vi "LSCI_4-28.vi"() -> ()   [LabVIEW 2019]
uses:
  <resource>/objmgr/daqmx.rc
  <vilib>/DAQmx/configure/timing.llb/DAQmx Timing (Sample Clock).vi
  <vilib>/DAQmx/create/channels.llb/DAQmx Create Channel (AO-Voltage-Basic).vi
  Settings.ctl
  <vilib>/DAQmx/write.llb/DAQmx Write (Digital 1D U32 1Chan NSamp).vi
  <vilib>/DAQmx/configure/trigger.llb/DAQmx Start Trigger (Digital Edge).vi
  <vilib>/DAQmx/write.llb/DAQmx Write (Analog DBL 1Chan 1Samp).vi
  <vilib>/DAQmx/read.llb/DAQmx Read (Counter DBL 1Chan 1Samp).vi
  <vilib>/DAQmx/create/channels.llb/DAQmx Create Channel (CI-Count Edges).vi
  <vilib>/DAQmx/create/channels.llb/DAQmx Create Channel (CO-Pulse Generation-Time).vi
  <vilib>/DAQmx/write.llb/DAQmx Write (Analog Wfm 1Chan NSamp).vi
  <vilib>/DAQmx/create/channels.llb/DAQmx Create Channel (DO-Digital Output).vi
  Control 2.ctl
panel:
  out "path":path=path "D:/Haad/v1.avi1.avi"
  in  "AVI Path 2":path=path "D:/Haad/v1.avi"
  in  "Trigger":bool
  in  "Color vs Monochrome":string="Y800 (720x540)"
  in  "ICImagingControl":refnum<k7>(container)
  in  "Grab":bool
  in  "Stop":bool
  in  "AOM Voltage":dbl=0.135 format="%0.3f"
  out "String 7":string="AOM Settings"
  out "String 6":string="Stroke Settings"
  out "String 5":string="Intrinsic Imaging"
  in  "LED 625 nm":bool
  in  "LED 580 nm":bool
  out "Trial #":i32=1
  out "Frames acquired":dbl=569.0 format="%0.2f"
  out "Number of Samples (Total)":dbl=10000.0
  out "Period (ms)":dbl=7.0
  out "String 4":string="Experimental Summary"
  out "String 3":string="Stimulation Control"
  out "String 2":string="Sequence Control"
  out "String":string="Trials Control"
  in  "Strength (V)":dbl=10.0
  in  "# of stimulations":i32=2
  in  "Delay (ms)":dbl=35.0
  in  "Width of pulse (ms)":dbl=70.0
  in  "# of Sequences":dbl=100.0
  in  "Delay End (ms)":i32=51
  in  "Sampling Rate (Hz)":T1=100000.0 format="%#_9f"
  in  "Frames/Seq":i32=7
  in  "Exposure Width (ms)":T1=5.0 format="%#_9f"
  in  "Time Between (ms)":T2=2.0 format="%#_9f"
  in  "Pre-stimulus Time":dbl=5.0 format="%.6f"
  in  "Time b/w Trials (s)":dbl=5.0 caption="Delay Time (s)"
  in  "# Trials":i32=2
  in  "Time domain signal":enum32{"Trigger Sequence", "Stimulation pulse"}(tab)=enum."Stimulation pulse"
  out "LSCI Sequence":cluster{i32, dbl, dbl[]}(graph)={0, 1e-05, array[10000 elements]}
  out "Whisker Stimulus Pulse":cluster{dbl[], dbl[]}(graph)
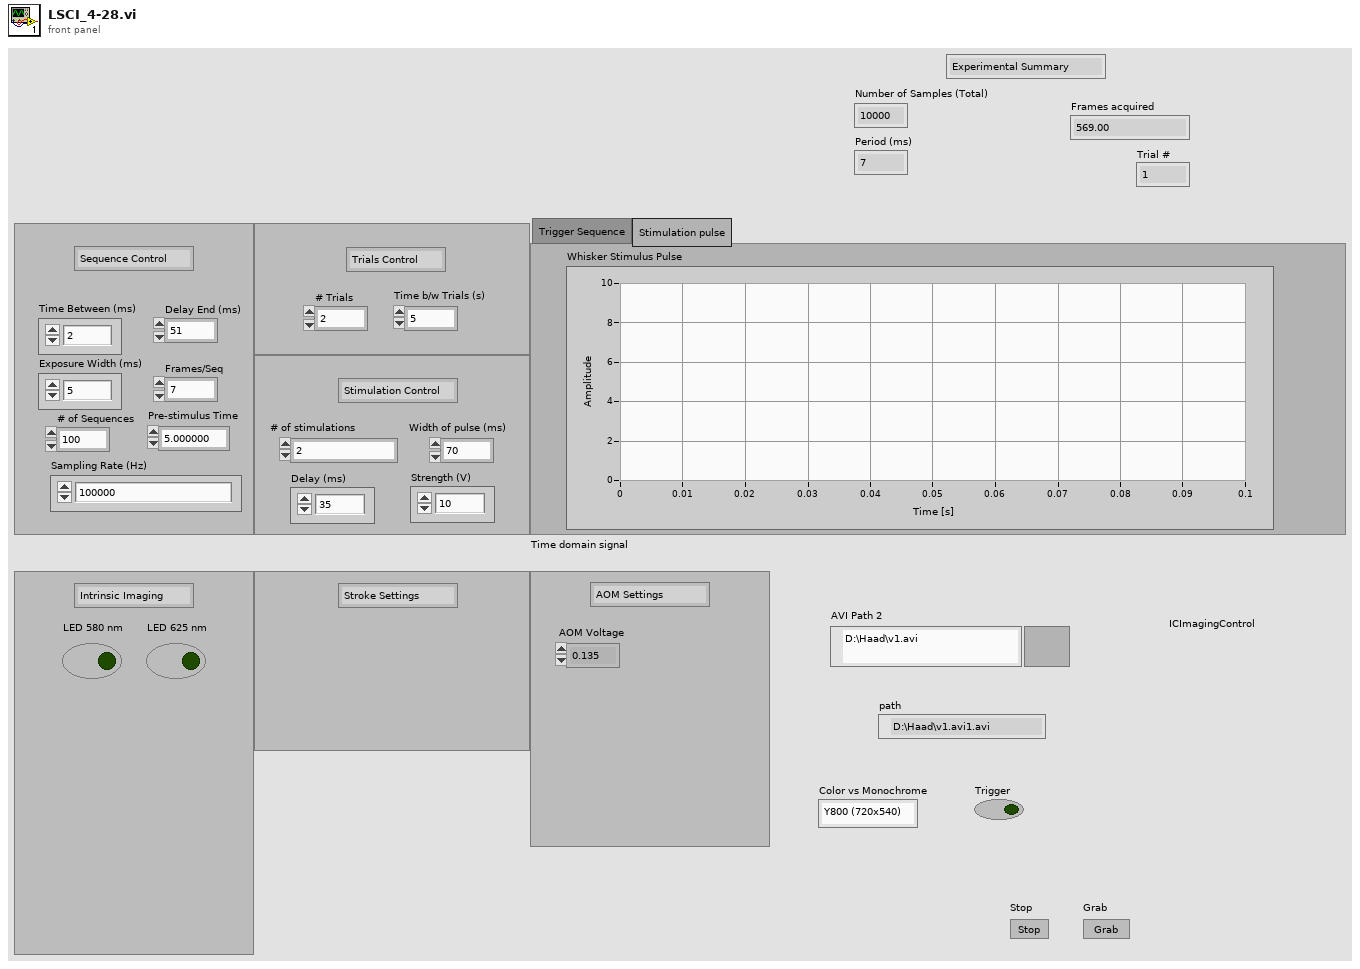
[diagram p1: front panel]
types:
  T1 = typedef "Settings.ctl" = dbl
  T2 = typedef "Control 2.ctl" = dbl
  T3 = typedef "IMAQ AVI2 Refnum.ctl" = refnum<k20>
  T4 = typedef "IMAQ Image.ctl" = refnum<image>
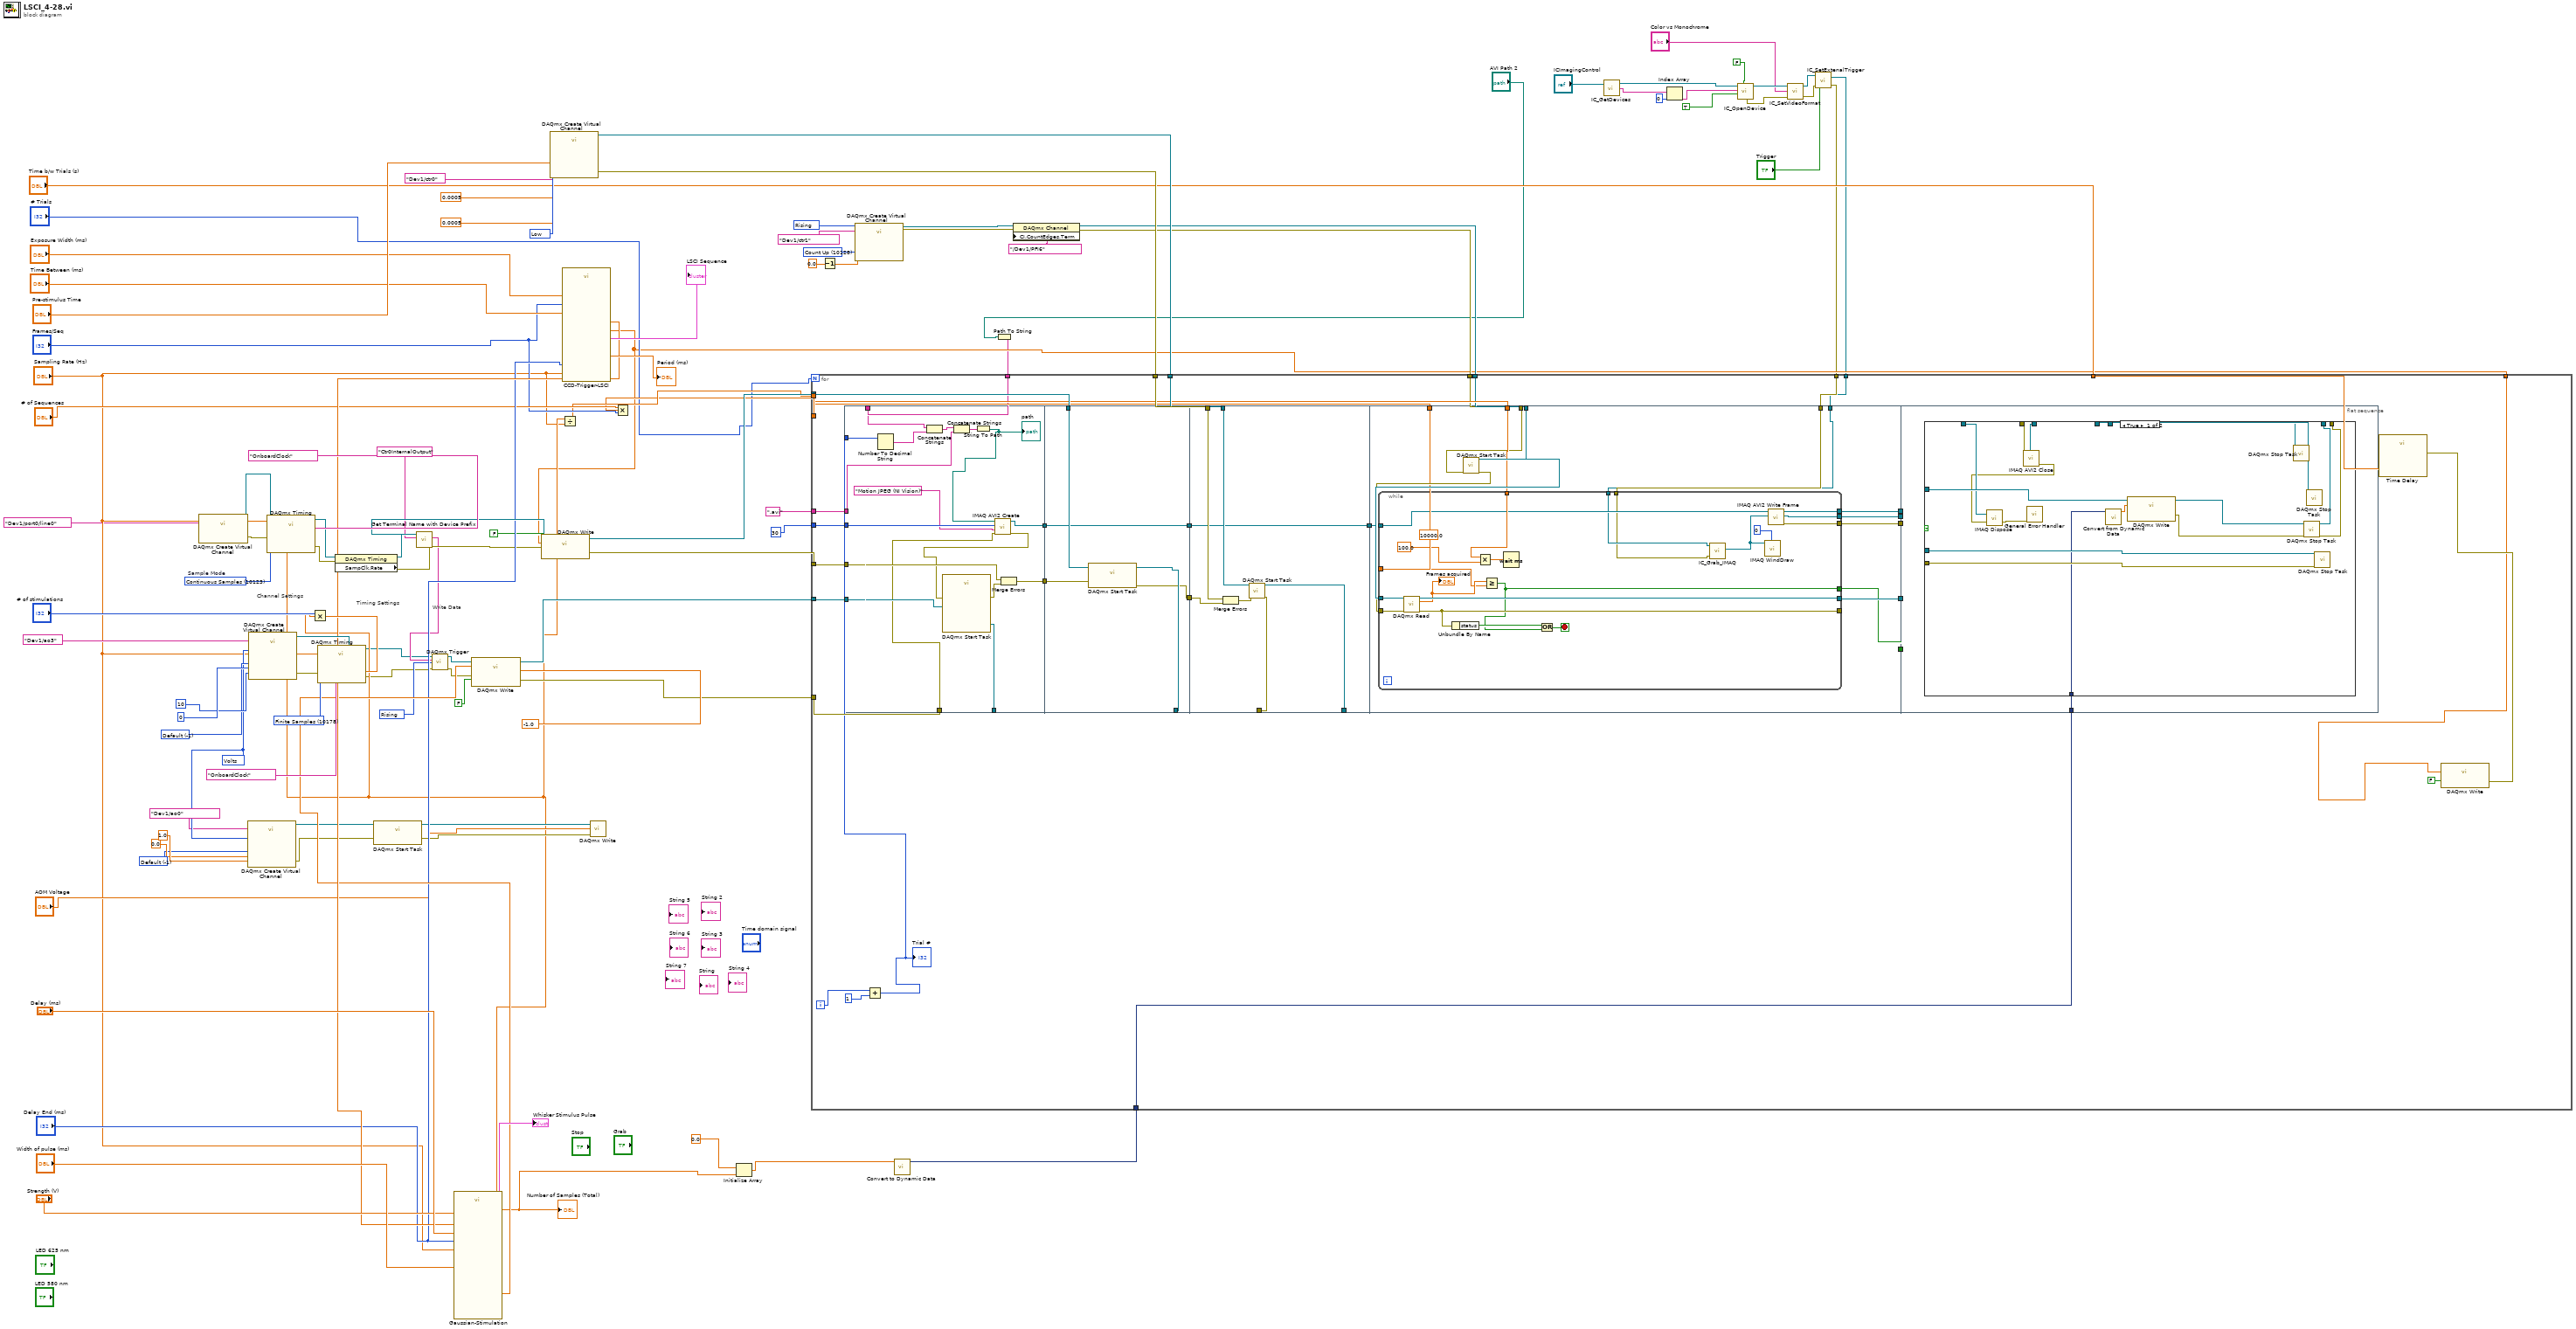
[diagram p0: block diagram]
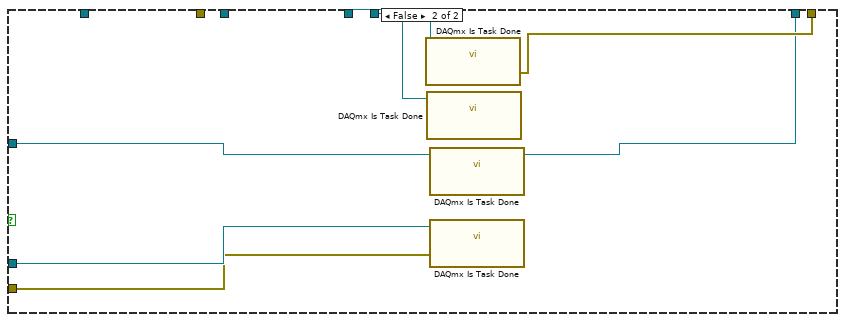
[diagram p2: hidden frame]
diagram:
  w24 = 10280 items=["Rising"=10280, "Falling"=10171] ("edge")
  w43 = -1 items=["Default"=-1, "RSE"=10083, "Differential"=10106, "Pseudodifferential"=12529] ("output terminal configuration")
  w61 = 10280 items=["Rising"=10280, "Falling"=10171] ("edge")
  w65 = 10128 items=["Count Up"=10128, "Count Down"=10124, "Externally Controlled"=10326] ("count direction")
  w91 = 10214 items=["High"=10192, "Low"=10214] ("Idle State")
  w98 = 10178 items=["Finite Samples"=10178, "Continuous Samples"=10123] ("sample mode")
  w99 = -1 items=["Default"=-1, "RSE"=10083, "Differential"=10106, "Pseudodifferential"=12529] ("output terminal configuration")
  w45 = 10348 items=["Volts"=10348, "From Custom Scale"=10065] ("units")
  w104 = 10123 items=["Finite Samples"=10178, "Continuous Samples"=10123, "Hardware Timed Single Point"=12522]  # Sample Mode
  # "Timing Settings"
  # "Write Data"
  # "Channel Settings"
  n1 = call-poly <vilib>:"DAQmx Create Virtual Channel.vi"("lines"=tag "Dev1/port0/line0") -> ("task out"=w27:refnum<k21>, "error out"=w79:errorcluster)  [unwired: 13 in]
  n2 = call-poly <vilib>:"DAQmx Create Virtual Channel.vi"("maximum value"=1.0, "minimum value"=0.0, "output terminal configuration"=w43, "physical channels"=tag "Dev1/ao0", "units"=w45) -> ("task out"=w38:refnum<k21>, "error out"=w37:errorcluster)  [unwired: 9 in]
  n3 = call-poly <vilib>:"DAQmx Create Virtual Channel.vi"("maximum value"=10, "minimum value"=0, "output terminal configuration"=w99, "physical channels"=tag "Dev1/ao3", "units"=w45) -> ("task out"=w96:refnum<k21>, "error out"=w97:errorcluster)  [unwired: 9 in]
  n4 = call <vilib>:"DAQmx Start Task.vi"("task/channels in"=w38, "error in"=w37) -> ("task out"=w36:refnum<k21>, "error out"=w35:errorcluster)  [unwired: 12 in]
  n5 = call-poly <vilib>:"DAQmx Create Virtual Channel.vi"("high time"=0.0005 ("High Time"), "low time"=0.0005 ("Low Time"), "counter"=tag "Dev1/ctr0" ("Counter(s)"), "idle state"=w91, "initial delay"="Pre-stimulus Time") -> ("task out"=w54:refnum<k21>, "error out"=w55:errorcluster)  [unwired: 4 in, 5 out]
  n6 = call "CCD-Trigger-LSCI.vi"("Sampling Rate"="Sampling Rate (Hz)", "Delay End (ms)"="Delay End (ms)", "Time Between (ms)"="Time Between (ms)", "Exposure Width (ms) in"="Exposure Width (ms)", "Frames/Seq"="Frames/Seq") -> ("# Samples"=w74:T1, "Period (ms)"=→"Period (ms)":dbl, "Array out"=w20:dbl[], "LSCI Sequence"=→"LSCI Sequence":cluster{i32, dbl, dbl[]})  [unwired: 2 in, 1 out]
  n7 = call "Gaussian-Stimulation.vi"("Strength (V)"="Strength (V)", "Delay (ms)"="Delay (ms)", "# Samples in"=w74, "Width of pulse (ms)"="Width of pulse (ms)", "Delay End (ms)"="Delay End (ms)", "Sampling Rate"="Sampling Rate (Hz)") -> ("Number of Samples (Total)"=w42:dbl, "Array 2"=w73:T1[], "# Samples out"=w30:T1, "Whisker Stimulus Pulse"=→"Whisker Stimulus Pulse":cluster{dbl[], dbl[]})  [unwired: 1 in, 1 out]
  "Number of Samples (Total)" <- w42
  n8 = call-poly <vilib>:"DAQmx Timing.vi"("task/channels in"=w27, "sample mode"=w104, "samples per channel"=w30, "rate"="Sampling Rate (Hz)", "source"=tag "OnboardClock", "error in"=w79) -> ("task out"=w31:refnum<k21>, "error out"=w32:errorcluster)  [unwired: 8 in]
  n9 = Multiply(x="# of stimulations", y=w30) -> (x*y=w85:T1)
  n10 = call-poly <vilib>:"DAQmx Timing.vi"("task/channels in"=w96, "sample mode"=w98, "samples per channel"=w85, "rate"="Sampling Rate (Hz)", "source"=tag "OnboardClock", "error in"=w97) -> ("task out"=w25:refnum<k21>, "error out"=w23:errorcluster)  [unwired: 1 in, 7 out]
  n11 = property class="DAQmx Timing" props=["SampClk.Rate"](reference=w31, error in=w32) -> (reference out=w95:refnum<k21>, error out=w71:errorcluster)  [unwired: 1 out]
  n12 = call "Get Terminal Name with Device Prefix.vi"("error in (no error)"=w71, "Local Terminal Name"="Ctr0InternalOutput" ("terminal"), "task/channels in"=w95) -> ("Terminal Name with Device Prefix"=w26:tag, "task out"=w94:refnum<k21>)  [unwired: 1 in, 6 out]
  n13 = call-poly <vilib>:"DAQmx Trigger.vi"("task/channels in"=w25, "source"=w26, "edge"=w24, "error in"=w23) -> ("task out"=w21:refnum<k21>, "error out"=w22:errorcluster)  [unwired: 1 in, 9 out]
  n14 = call-poly <vilib>:"DAQmx Write.vi"("task/channels in"=w21, "auto start"=FALSE, "data"=w73, "timeout"=-1.0 ("Wirite Timeout"), "error in"=w22) -> ("task out"=w33:refnum<k21>, "error out"=w57:errorcluster)  [unwired: 9 out]
  n15 = call-poly <vilib>:"DAQmx Write.vi"("task/channels in"=w94, "auto start"=FALSE, "data"=w20, "error in"=w71) -> ("task out"=w56:refnum<k21>, "error out"=w58:errorcluster)  [unwired: 9 in, 1 out]
  n16 = Divide(x=w30, y="Sampling Rate (Hz)") -> (x/y=w53:T1)
  n17 = call-poly <vilib>:"DAQmx Write.vi"("task/channels in"=w36, "data"="AOM Voltage", "error in"=w35) -> ()  [unwired: 10 in, 3 out]
  n18 = Multiply(x="# of Sequences", y="Frames/Seq") -> (x*y=w52:dbl)
  n19 = Initialize Array(0.0 ("element"), w42) -> (w40:dbl[])
  n20 = Decrement(x=0.0) -> (x-1=w64:dbl)
  n21 = call-poly <vilib>:"DAQmx Create Virtual Channel.vi"("initial count"=w64, "count direction"=w65, "edge"=w61, "counter"=tag "Dev1/ctr1") -> ("task out"=w62:refnum<k21>, "error out"=w63:errorcluster)  [unwired: 10 in]
  n22 = call "Convert to Dynamic Data"("Array"=w40) -> ("Dynamic Data Type"=w39:dynamicdata)  [unwired: 3 in]
  n23 = Path To String(path="AVI Path 2") -> (string=w3:string)
  n24 = property class="DAQmx Channel"(reference=w62, error in=w63, "CI.CountEdges.Term"=tag "/Dev1/PFI6") -> (reference out=w51:refnum<k21>, error out=w50:errorcluster)
  n25 = call <userlib>:"IC_GetDevices.vi"("ICImagingControl In"="ICImagingControl") -> ("ICImagingControl Out"=w16:refnum<k7>, "Devices"=w15:string[])  [unwired: 1 in, 1 out]
  n26 = Index Array(array=w15, index=0) -> (element=w13:string)
  n27 = call <userlib>:"IC_OpenDevice.vi"("Color"=FALSE, "Live"=TRUE, "Device"=w13, "ICImagingControl In"=w16) -> ("ICImagingControl Out"=w12:refnum<k7>, "Error Out"=w10:errorcluster)  [unwired: 2 in, 4 out]
  n28 = call <userlib>:"IC_SetVideoFormat.vi"("Error In (no error)"=w10, "VideoFormat"="Color vs Monochrome", "ICImagingControl In"=w12) -> ("Error Out"=w7:errorcluster, "ICImagingControl Out"=w9:refnum<k7>)  [unwired: 1 out]
  n29 = call <userlib>:"IC_SetExtenalTrigger.vi"("Error In (no error)"=w7, "Trigger"="Trigger", "ICImagingControl In"=w9) -> ("Error Out"=w6:errorcluster, "ICImagingControl Out"=w5:refnum<k7>)
  n30 = for {
    N: "# Trials" -> [_]
    tunnel: w58 -> [w140]
    tunnel: w33 -> [w139]
    tunnel: w57 -> [w138]
    tunnel: w56 -> [w136]
    tunnel: w55 -> [w134]
    tunnel: w54 -> [w133]
    tunnel: w53 -> [w131]
    tunnel: w52 -> [w130]
    tunnel: w51 -> [w129]
    tunnel: w50 -> [w128]
    tunnel: "Time b/w Trials (s)" -> [w125]
    tunnel: w39 -> [w105]
    tunnel: w20 -> [w120]
    tunnel: w6 -> [w119]
    tunnel: w5 -> [w118]
    tunnel: w3 -> [w116]
    tunnel: ".avi" ("string") -> [w115]
    tunnel: u32 30 ("Frames Per Second") -> [w114]
    i -> [w127]
    n31 = flat-sequence {
      tunnel: w140 -> [w158]
      tunnel: w139 -> [w157]
      tunnel: w138 -> [w146]
      tunnel: [w156] -> w137
      tunnel: [w155] -> w142
      tunnel: w117 -> [w154]
      tunnel: w116 -> [w152]
      tunnel: w115 -> [w150]
      tunnel: w114 -> [w147]
      tunnel: [w143] -> w111
      tunnel: w136 -> [w164]
      tunnel: [w163] -> w135
      tunnel: w142 -> [w162]
      tunnel: [w161] -> w141
      tunnel: [w160] -> w112
      tunnel: w111 -> [w160]
      tunnel: w134 -> [w170]
      tunnel: w133 -> [w169]
      tunnel: [w168] -> w132
      tunnel: w141 -> [w167]
      tunnel: [w166] -> _
      tunnel: [w165] -> w113
      tunnel: w112 -> [w165]
      tunnel: w131 -> [w183]
      tunnel: w130 -> [w182]
      tunnel: w129 -> [w181]
      tunnel: w128 -> [w180]
      tunnel: w119 -> [w177]
      tunnel: w118 -> [w176]
      tunnel: w113 -> [w175]
      tunnel: [w178] -> w110
      tunnel: [w179] -> w109
      tunnel: [w174] -> w108
      tunnel: [w173] -> w107
      tunnel: [w172] -> w106
      tunnel: w110 -> [_]
      tunnel: w109 -> [_]
      tunnel: w108 -> [_]
      tunnel: w107 -> [_]
      tunnel: w106 -> [_]
      tunnel: w105 -> [w206]
      frame #0 {
        n32 = Number To Decimal String(number=w154) -> (decimal integer string=w153:string)  [unwired: 1 in]
        n33 = Concatenate Strings(w152, w153) -> (w151:string)
        n34 = Concatenate Strings(w151, w150) -> (w149:string)
        n35 = String To Path(string=w149) -> (path=w148:path)
        "path" <- w148
        n36 = call "IMAQ AVI2 Create"("error in (no error)"=w146, "Codec"="Motion JPEG (NI Vision)", "Frames Per Second"=w147, "AVI Path"=w148) -> ("error out"=w145:errorcluster, "AVI Refnum"=w143:T3)  [unwired: 6 in]
        n37 = call <vilib>:"DAQmx Start Task.vi"("task/channels in"=w157, "error in"=w145) -> ("task out"=w156:refnum<k21>, "error out"=w159:errorcluster)  [unwired: 12 out]
        n38 = Merge Errors(w158, w159) -> (w155:errorcluster)
      }
      frame #1 {
        n39 = call <vilib>:"DAQmx Start Task.vi"("task/channels in"=w164, "error in"=w162) -> ("task out"=w163:refnum<k21>, "error out"=w161:errorcluster)  [unwired: 12 in]
      }
      frame #2 {
        n40 = Merge Errors(w170, w167) -> (w171:errorcluster)
        n41 = call <vilib>:"DAQmx Start Task.vi"("task/channels in"=w169, "error in"=w171) -> ("task out"=w166:refnum<k21>, "error out"=w168:errorcluster)  [unwired: 12 out]
      }
      frame #3 {
        n42 = call <vilib>:"DAQmx Start Task.vi"("task/channels in"=w181, "error in"=w180) -> ("task out"=w185:refnum<k21>, "error out"=w184:errorcluster)  [unwired: 12 in]
        n43 = while {
          tunnel: w185 -> [w205]
          tunnel: w184 -> [w204]
          tunnel: [w203] -> w179
          tunnel: [w202] -> _
          tunnel: w183 -> [w201]
          tunnel: w182 -> [w197]
          tunnel: [w194] -> w178
          tunnel: w177 -> [w191]
          tunnel: w176 -> [w192]
          tunnel: w175 -> [w193]
          tunnel: [w190] -> w174
          tunnel: [w189] -> w173
          tunnel: [w188] -> w172
          stop <- w195 stop-if-true
          (unwired) T1 10000.0 ("y")
          n44 = call-poly <vilib>:"DAQmx Read.vi"("task/channels in"=w205, "error in"=w204) -> ("task out"=w203:refnum<k21>, "data"=w198:dbl, "error out"=w202:errorcluster)  [unwired: 11 in]
          "Frames acquired" <- w198
          n45 = Unbundle By Name(w202) -> ("status"=w196:bool)
          n46 = Multiply(x=w201, y=T1 100.0) -> (x*y=w200:T1)
          n47 = Greater Or Equal?(x=w198, y=w197) -> (x >= y?=w194:bool)
          n48 = Wait (ms)(milliseconds to wait=w200) -> ()  [unwired: 1 out]
          n49 = Or(x=w196, y=w194) -> (x .or. y?=w195:bool)
          n50 = call <userlib>:"IC_Grab_IMAQ.vi"("ICImagingControl In"=w192, "Error In (no error)"=w191) -> ("Image Out"=w187:T4)  [unwired: 1 in, 3 out]
          n51 = call "IMAQ WindDraw"("Window Number (0...15)"=0, "Image"=w187) -> ()  [unwired: 8 in, 2 out]
          n52 = call "IMAQ AVI2 Write Frame"("Image"=w187, "AVI Refnum"=w193) -> ("error out"=w189:errorcluster, "Image Out (duplicate)"=w188:T4, "AVI Refnum (duplicate)"=w190:T3)  [unwired: 7 in]
        }
      }
      frame #4 {
        n53 = case shown="True" {
          selector: _ -> [_ _]
          tunnel: _ -> [w218 w227]
          tunnel: _ -> [w219 w228]
          tunnel: _ -> [w220 w229]
          tunnel: _ -> [w222 w226]
          tunnel: [w214 w225] -> _
          tunnel: _ -> [w221 w224]
          tunnel: [w213 w223] -> _
          tunnel: _ -> [w212 _]
          tunnel: _ -> [w211 _]
          tunnel: _ -> [w209 _]
          tunnel: w206 -> [w207 _]
          frame True {
            n54 = call "IMAQ AVI2 Close"("error in (no error)"=w211, "AVI Refnum"=w212) -> ("error out"=w208:errorcluster)  [unwired: 9 in]
            n55 = call "IMAQ Dispose"("Image"=w209, "error in (no error)"=w208) -> ("error out"=w210:errorcluster)  [unwired: 4 in]
            n56 = call <vilib>:"General Error Handler.vi"("error in (no error)"=w210) -> ()  [unwired: 10 in, 5 out]
            n57 = call "Convert from Dynamic Data"("Dynamic Data Type"=w207) -> ("Array"=w217:dbl[])  [unwired: 3 in]
            n58 = call-poly <vilib>:"DAQmx Write.vi"("task/channels in"=w218, "data"=w217) -> ("task out"=w216:refnum<k21>, "error out"=w215:errorcluster)  [unwired: 11 in, 1 out]
            n59 = call <vilib>:"DAQmx Stop Task.vi"("task/channels in"=w221) -> ()  [unwired: 13 in, 2 out]
            n60 = call <vilib>:"DAQmx Stop Task.vi"("task/channels in"=w216, "error in"=w215) -> ("task out"=w213:refnum<k21>, "error out"=w214:errorcluster)  [unwired: 12 in]
            n61 = call <vilib>:"DAQmx Stop Task.vi"("task/channels in"=w222) -> ()  [unwired: 13 in, 2 out]
            n62 = call <vilib>:"DAQmx Stop Task.vi"("task/channels in"=w220, "error in"=w219) -> ()  [unwired: 12 in, 2 out]
          }
          frame False {
            n63 = call <vilib>:"DAQmx Is Task Done.vi"("task/channels in"=w226) -> ("error out"=w225:errorcluster)  [unwired: 12 in, 2 out]
            n64 = call <vilib>:"DAQmx Is Task Done.vi"("task/channels in"=w224) -> ()  [unwired: 12 in, 3 out]
            n65 = call <vilib>:"DAQmx Is Task Done.vi"("task/channels in"=w227) -> ("task out"=w223:refnum<k21>)  [unwired: 12 in, 2 out]
            n66 = call <vilib>:"DAQmx Is Task Done.vi"("task/channels in"=w229, "error in"=w228) -> ()  [unwired: 11 in, 3 out]
          }
        }
      }
    }
    n67 = Add(x=w127, y=1) -> (x+y=w117:i32)
    "Trial #" <- w117
    n68 = call-poly <vilib>:"DAQmx Write.vi"("auto start"=FALSE, "data"=w120) -> ("task/channels in"=w122:refnum<k21>, "error in"=w124:errorcluster, "error out"=w121:errorcluster)  [unwired: 9 in, 2 out]
    n69 = call "Time Delay"("error in (no error)"=w121, "Delay Time (s)"=w125) -> ()  [unwired: 9 in, 1 out]
  }
